vi "Outputs.vi"(8 "error in (no error)":errorcluster, 11 "Agitator Module State Cluster":T1={"State"=enum."Idle", "Start Time"=timestamp(0 s since 1904-01-01), "Current Time"=timestamp(0 s since 1904-01-01), "Agitator Module Config"={"GUID"="", "Drop Coords"={"Horizontal"=0, "Vertical"=0}, "Process Name"="", "User name"="", "Queue Name"="", "Settings"={"Cycle Period"=500.0, "Agitator Type"="", "Setpoint (µm)"=0.0, "IKA EUROSTAR Settings"={"VISA resource name"="", "Simulated?"=FALSE}}, "Load Count"=0}, "Output Error"=FALSE, "Log Started"=FALSE, "First Iteration"=FALSE, "Data"={"Agitator rpm Value"=0.0}, "Agitator On?"=enum."Off"}) -> (0 "error out":errorcluster, 3 "Agitator Module State Cluster":T1={"State"=enum."Idle", "Start Time"=timestamp(0 s since 1904-01-01), "Current Time"=timestamp(0 s since 1904-01-01), "Agitator Module Config"={"GUID"="", "Drop Coords"={"Horizontal"=0, "Vertical"=0}, "Process Name"="", "User name"="", "Queue Name"="", "Settings"={"Cycle Period"=500.0, "Agitator Type"="", "Setpoint (µm)"=0.0, "IKA EUROSTAR Settings"={"VISA resource name"="", "Simulated?"=FALSE}}, "Load Count"=0}, "Output Error"=FALSE, "Log Started"=FALSE, "First Iteration"=FALSE, "Data"={"Agitator rpm Value"=0.0}, "Agitator On?"=enum."Off"})   [LabVIEW 2018, in "Agitator Module.lvlib" / "Agitator Module Engine.lvlib"]
uses:
  Agitator Module Engine.lvlib
  Feed Module/Controls/Agitator Module State Cluster.ctl
  Pump Module Folder/Measure Instrument/State Enum.ctl
  Feed Module/Controls/Agitator Module Config Cluster.ctl
  <vilib>/Utility/miscctls.llb/LVPoint32TypeDef.ctl
  Feed Module/Controls/Agitator Module Settings Cluster.ctl
  IKA EUROSTAR/IKA EUROSTAR Settings.ctl
  Tag VIs/Tag FGV Operation Enum.ctl
  Shared Variables/Dynamic Shared Variables.lvlib
  Sonic Systems P100/Sonic Systems P100.lvlib
  Agitator Module.lvlib
  Pump Module Folder/Measure Instrument/Pump Module Engine.lvlib
  IKA EUROSTAR/IKA EUROSTAR.lvlib
panel:
  # "Agitator Settings"
  # "Agitator Settings"
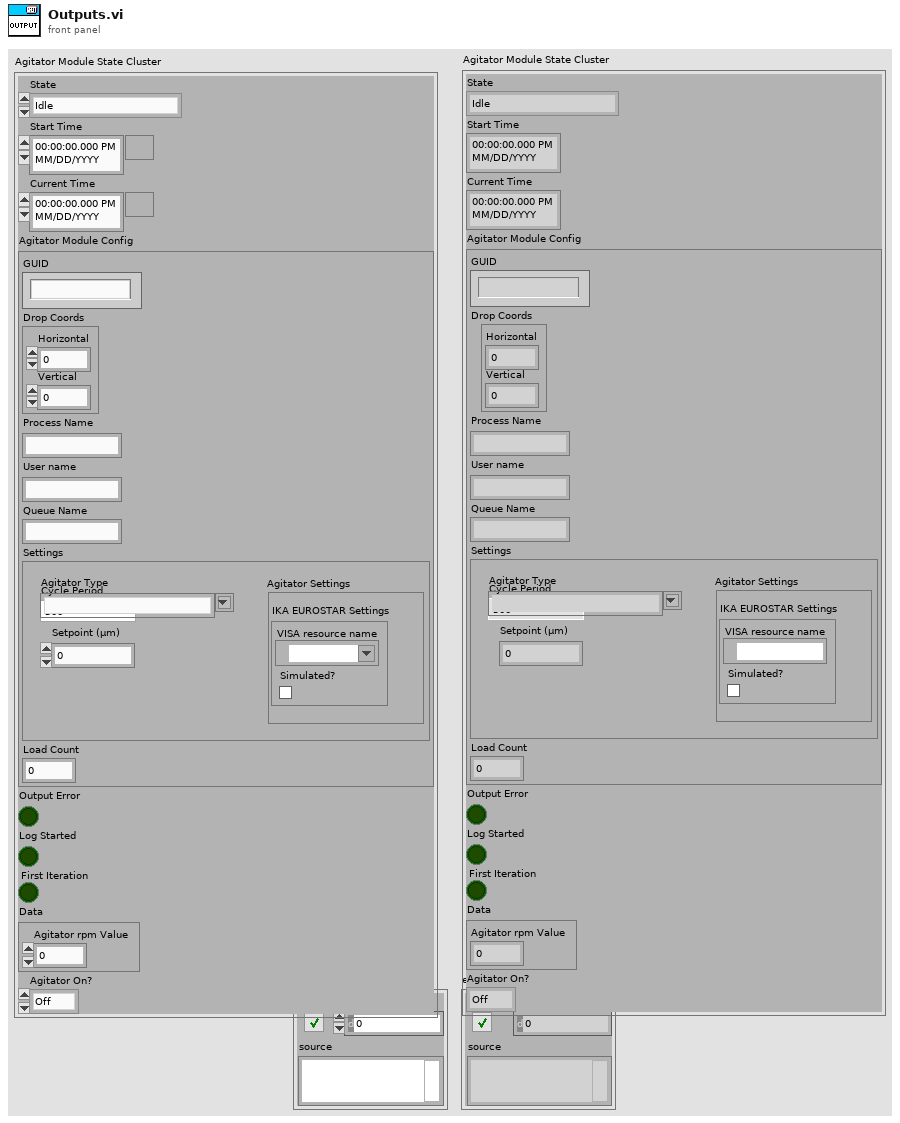
[diagram p1: front panel]
types:
  T1 = typedef "Agitator Module.lvlib/Agitator Module State Cluster.ctl" = cluster{"State":T2, "Start Time":timestamp, "Current Time":timestamp, "Agitator Module Config":T3, "Output Error":bool, "Log Started":bool, "First Iteration":bool, "Data":cluster{"Agitator rpm Value":dbl}, "Agitator On?":enum16{"Off", "On", "Not Initialized", "Over Cutoff"}}
  T2 = typedef "Pump Module.lvlib/Pump Module Engine.lvlib/State Enum.ctl" = enum16{"Measuring", "Idle", "Paused"}
  T3 = typedef "Agitator Module.lvlib/Agitator Module Config Cluster.ctl" = cluster{"GUID":string, "Drop Coords":T4, "Process Name":string, "User name":string, "Queue Name":string, "Settings":T5, "Load Count":i32}
  T4 = typedef "LVPoint32TypeDef.ctl" = cluster{"Horizontal":i32, "Vertical":i32}
  T5 = typedef "Agitator Module.lvlib/Agitator Module Settings Cluster.ctl" = cluster{"Cycle Period":dbl, "Agitator Type":string, "Setpoint (µm)":dbl, "IKA EUROSTAR Settings":T6}
  T6 = typedef "IKA EUROSTAR.lvlib/IKA EUROSTAR Settings.ctl" = cluster{"VISA resource name":refnum<visa-resource-name>, "Simulated?":bool}
  T7 = typedef "Tag FGV Operation Enum.ctl" = enum16{"Init", "Set Notification Queue", "Create Tag", "Commit", "Write Tag (Numeric)", "Write Tag (Boolean)", "Read All Tags", "Read One Tag", "Delete Tag Category", "Set Alarm Parameters (Numeric)", "Set Alarm Parameters (Boolean)", "Enable All Alarms", "Disable All Alarms", "Delete All Tags", "Read Alarms", "Ack Alarm", "Read Alarm Parameters (Numeric)", "Read Alarm Parameters (Boolean)"}
  T8 = cluster{"Amplitude Tag":string, "Power Tag":string, "Output Device Tag":string}
  T9 = enum16{"Off", "On", "Not Initialized", "Over Cutoff"}
  T10 = typedef "Sonic Systems P100.lvlib/Sonic Systems P100 Settings.ctl" = cluster{"VISA resource name":refnum<visa-resource-name>, "Simulated?":bool}
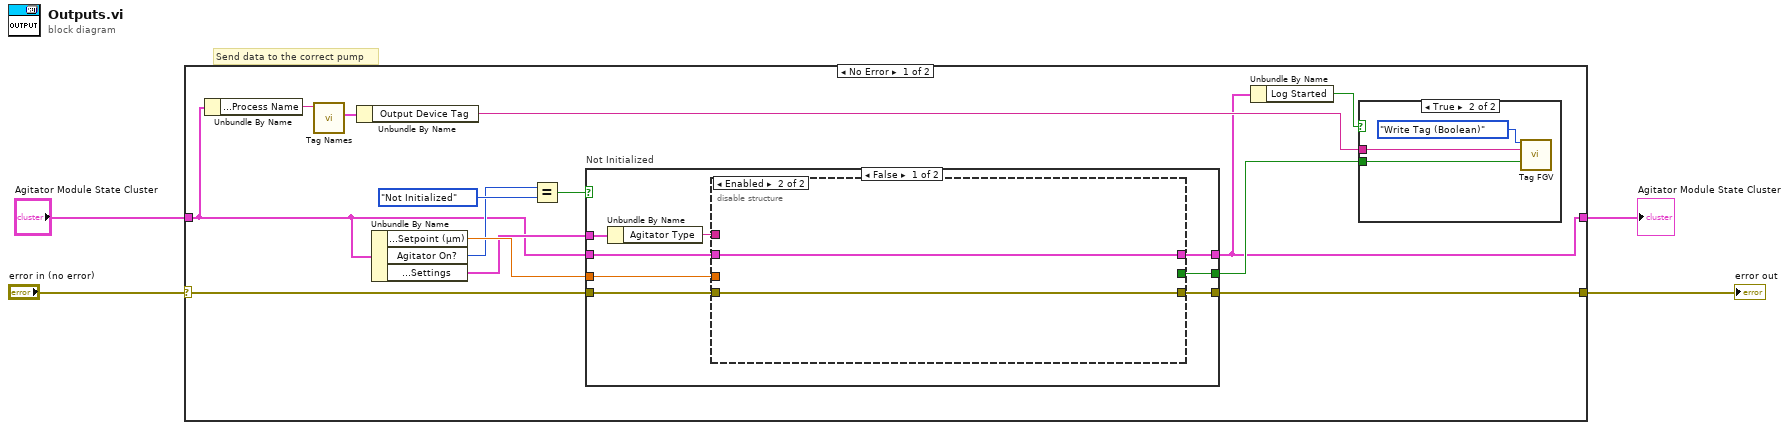
[diagram p0: block diagram]
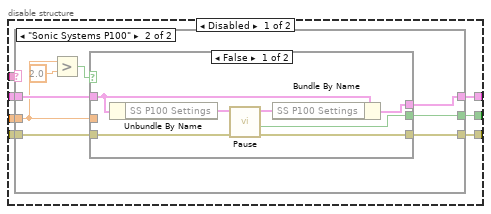
[diagram p3: hidden frame]
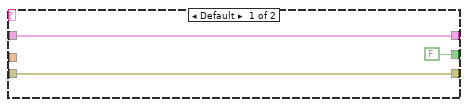
[diagram p4: hidden frame]
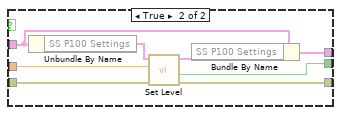
[diagram p5: hidden frame]
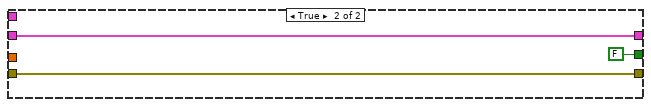
[diagram p6: hidden frame]
diagram:
  # "Send data to the correct pump"
  n1 = case shown="No Error" "error in (no error)" {
    selector: "error in (no error)" -> [w18 w69]
    tunnel: [w17 w69] -> w3
    tunnel: "Agitator Module State Cluster" -> [w5 w68]
    tunnel: [w11 w68] -> w1
    frame No Error {
      n2 = Unbundle By Name(w5) -> ("Agitator Module Config.Process Name"=w7:string)
      n3 = call "Tag Names.vi"("Process Name"=w7) -> ("SC Tags"=w8:T8)  [unwired: 8 in, 2 out]
      n4 = Unbundle By Name(w8) -> ("Output Device Tag"=w16:string)
      n5 = Unbundle By Name(w5) -> ("Agitator Module Config.Settings.Setpoint (µm)"=w12:dbl, "Agitator On?"=w9:T9, "Agitator Module Config.Settings"=w6:T5)
      n6 = Equal?(x=w9, y=enum16{"Off", "On", "Not Initialized"}."Not Initialized" ("x")) -> (x = y?=w14:bool)
      n7 = case "Not Initialized" shown="False" w14 {
        tunnel: w18 -> [w26 w66]
        tunnel: [w25 w66] -> w17
        tunnel: [w22 FALSE ("Connection Error")] -> w15
        tunnel: w12 -> [w24 _]
        tunnel: [w27 w65] -> w11
        tunnel: w6 -> [w29 _]
        tunnel: w5 -> [w23 w65]
        frame False {
          n8 = Unbundle By Name(w29) -> ("Agitator Type"=w28:string)
          n9 = disable-structure shown="Enabled" {
            disable-tunnel: w28 -> [w36 _]
            disable-tunnel: [w35 w64] -> w27
            disable-tunnel: w26 -> [w34 w63]
            disable-tunnel: [w33 w63] -> w25
            disable-tunnel: w24 -> [w32 _]
            disable-tunnel: w23 -> [w31 w64]
            disable-tunnel: [w30 _] -> w22
            frame Disabled {
              n10 = case shown="\"Sonic Systems P100\"" w36 {
                tunnel: [w37 w45] -> w35
                tunnel: w34 -> [w39 w47]
                tunnel: [w39 w44] -> w33
                tunnel: w32 -> [_ w42]
                tunnel: w31 -> [w37 w46]
                tunnel: [FALSE ("Connection Error") w43] -> w30
                frame Default {
                }
                frame "Sonic Systems P100" {
                  n11 = Greater?(x=w42, y=2.0) -> (0:w40:bool)
                  n12 = case shown="False" w40 {
                    tunnel: w47 -> [w54 w62]
                    tunnel: w42 -> [_ w61]
                    tunnel: w46 -> [w49 w59]
                    tunnel: [w48 w57] -> w45
                    tunnel: [w53 w56] -> w44
                    tunnel: [w52 w55] -> w43
                    frame False {
                      n13 = Unbundle By Name(w49) -> ("SS P100 Settings"=w50:T10)
                      n14 = call "Pause.vi"("error in (no error)"=w54, "SS P100 Settings In"=w50) -> ("error out"=w53:errorcluster, "Connection Error"=w52:bool, "SS P100 Settings Out"=w51:T10)  [unwired: 7 in]
                      n15 = Bundle By Name(cluster=w49, "SS P100 Settings"=w51) -> (w48:T1)
                    }
                    frame True {
                      n16 = Unbundle By Name(w59) -> ("SS P100 Settings"=w60:T10)
                      n17 = call "Set Level.vi"("error in (no error)"=w62, "Setpoint"=w61, "SS P100 Settings In"=w60) -> ("error out"=w56:errorcluster, "Connection Error"=w55:bool, "SS P100 Settings Out"=w58:T10)  [unwired: 6 in]
                      n18 = Bundle By Name(cluster=w59, "SS P100 Settings"=w58) -> (w57:T1)
                    }
                  }
                }
              }
            }
            frame Enabled {
            }
          }
        }
        frame True {
        }
      }
      n19 = Unbundle By Name(w11) -> ("Log Started"=w13:bool)
      n20 = case shown="True" w13 {
        tunnel: w16 -> [_ w21]
        tunnel: w15 -> [_ w20]
        frame False {
        }
        frame True {
          n21 = call "Tag FGV.vi"("Operation"=Tag_FGV_Operation_Enum."Write Tag (Boolean)", "Tag Name"=w21, "Data"=w20) -> ()  [unwired: 5 in, 8 out]
        }
      }
    }
    frame Error {
    }
  }
  "error out" <- w3
  "Agitator Module State Cluster" <- w1
